vi "sub_table_open.vi"() -> (0 "Cluster (Ausgang)":T1)   [LabVIEW 2009]
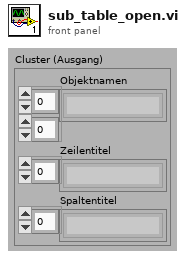
[diagram p1: front panel]
types:
  T1 = cluster{"Objektnamen":string[][], "Zeilentitel":string[], "Spaltentitel":string[]}
  T2 = enum16{"open", "replace", "create", "open or create", "replace or create", "replace or create with confirmation"}
  T3 = cluster{"[0]":string, "[1]":string, "[2]":string, "[3]":string, "[4]":string, "[5]":string, "[6]":string, "[7]":string, "[8]":string}
  T4 = cluster{"[0]":string, "[1]":string, "[2]":string, "[3]":string, "[4]":string, "[5]":string, "[6]":string, "[7]":string, "[8]":string}[]
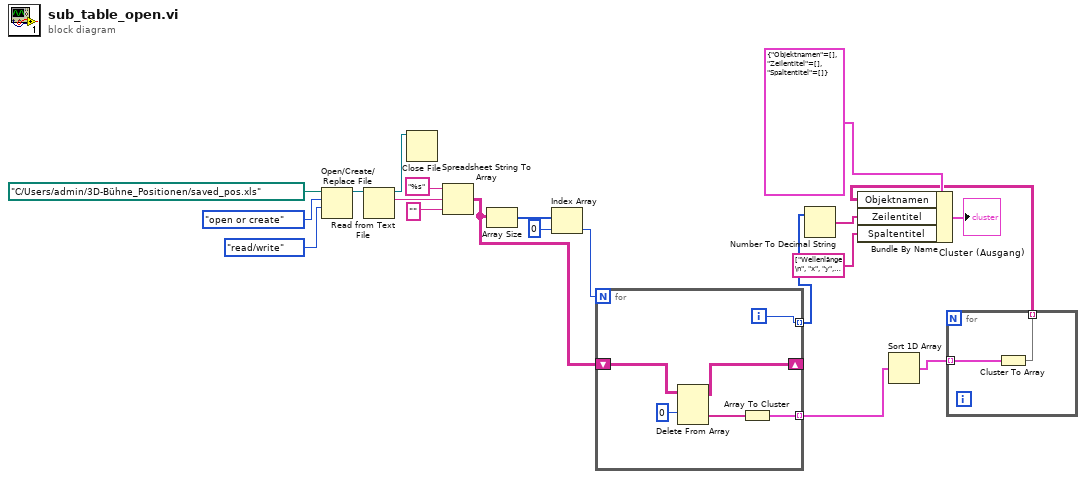
[diagram p0: block diagram]
diagram:
  n1 = Open/Create/Replace File(file path (use dialog)=path "C:/Users/admin/3D-Bühne_Positionen/saved_pos.xls" ("Dateipfad (Dialog verwenden)"), operation (0:open)=T2."open or create" ("Operation (0:Öffnen)"), access (0:read/write)=enum16{"read/write", "read-only", "write-only"}."read/write" ("Zugriff (0:Lesen/Schreiben)")) -> (refnum out=w17:refnum<file>)  [unwired: 3 in, 2 out]
  n2 = Read from Text File(file (use dialog)=w17) -> (refnum out=w14:refnum<file>, text=w20:string)  [unwired: 3 in, 2 out]
  n3 = Close File(refnum=w14) -> ()  [unwired: 1 in, 2 out]
  n4 = Spreadsheet String To Array(format string="%s" ("Format-String"), spreadsheet string=w20, array type (2D Dbl)="") -> (array=w5:string[][])  [unwired: 1 in]
  n5 = Array Size(array=w5) -> (size(s)=w13:i32[])
  n6 = Index Array(array=w13, index=0 ("Index")) -> (element=w11:i32)
  n7 = for {
    N: w11 -> [_]
    tunnel: [w26] -> w1 mode=indexing
    shift-right: [w24] -> _
    shift-left: w5 -> [w25]
    tunnel: [w21] -> w4 mode=indexing
    i -> [w26]
    n8 = Delete From Array(array=w25, index (row)=0 ("Index (Zeile)")) -> (deleted portion=w22:string[], array with subset deleted=w24:string[][])  [unwired: 2 in]
    n9 = Array To Cluster(array=w22) -> (cluster=w21:T3)
  }
  n10 = Number To Decimal String(number=w1) -> (decimal integer string=w8:string[])  [unwired: 1 in]
  n11 = Sort 1D Array(array=w4) -> (sorted array=w3:T4)
  n12 = for {
    tunnel: w3 -> [w28] mode=indexing
    tunnel: [w27] -> w2 mode=indexing
    n13 = Cluster To Array(cluster=w28) -> (array=w27:string[])
  }
  n14 = Bundle By Name(cluster=T1 {"Objektnamen"=[], "Zeilentitel"=[], "Spaltentitel"=[]}, "Objektnamen"=w2, "Zeilentitel"=w8, "Spaltentitel"=string[] ["Wellenlänge\n", "x", "y", "z", "Bemerkung"] ("Spaltentitel[]")) -> (→"Cluster (Ausgang)":T1)
